vi "Construct Logging.vi"(7 "timing channel offset (-1)":i64=-1, 8 "error in":errorcluster, 10 "Logging hardware channels in":T2[](array[typedef]) {"labels settings for RT"."Label Timestamp Channel Data Reference" format="%.0x"; "labels settings for RT"."Word Initial Raw Value" format="%032.0f"; "labels settings for RT"."Label Disable/Trigger Channel Reference" format="%.0x"; "labels settings for RT"."parameter driver data"."Tx parameter refs" format="%.0x"; "labels settings for RT"."SDI" format="%02b"; "labels settings for RT"."label" format="%.0o"}, 11 "custom device ref in":T1=18446744073709551615 format="%.0x") -> (0 "error out":errorcluster, 2 "Logging Execution Unit out":refnum<class "Logging Execution Unit.lvclass">, 3 "custom device ref out":T1=18446744073709551615 format="%.0x")   [LabVIEW 2020, in "AIM ARINC 429 Engine.lvlib" / "Implementation.lvlib" / "Logging Execution Unit.lvclass"]
uses:
  Logging Execution Unit.lvclass
  Execution Unit Factory/Execution Unit Factory.lvclass
  Execution Unit/Execution Unit.lvclass
  Scripting/AIM/AIM ARINC 429 Scripting.lvlib
  C:/Users/nitest/Desktop/Git 2020/niveristand-aim-arinc429-custom-device/Source/Custom Device Support/Engine/Implementation/Execution Unit/Execution Unit.lvclass
  Shared/Label.ctl
  <vilib>/NI/NI VeriStand Encoding and Decoding/Encoding.ctl
  <vilib>/NI/NI VeriStand Encoding and Decoding/Encoding and Decoding.lvlib
  Shared/Parameter Definition.ctl
  <vilib>/NI VeriStand/Custom Device API/Custom Device Item Ref.ctl
  <vilib>/NI VeriStand/Custom Device API/Custom Device API.lvlib
  Shared/RT Parameters.ctl
  Shared/Transfer Type.ctl
  <vilib>/NI VeriStand/Custom Device API/Data Reference.ctl
  Shared/RT Label Settings.ctl
  Shared/RT Hardware Channel Settings.ctl
  Shared/Transfer Speed.ctl
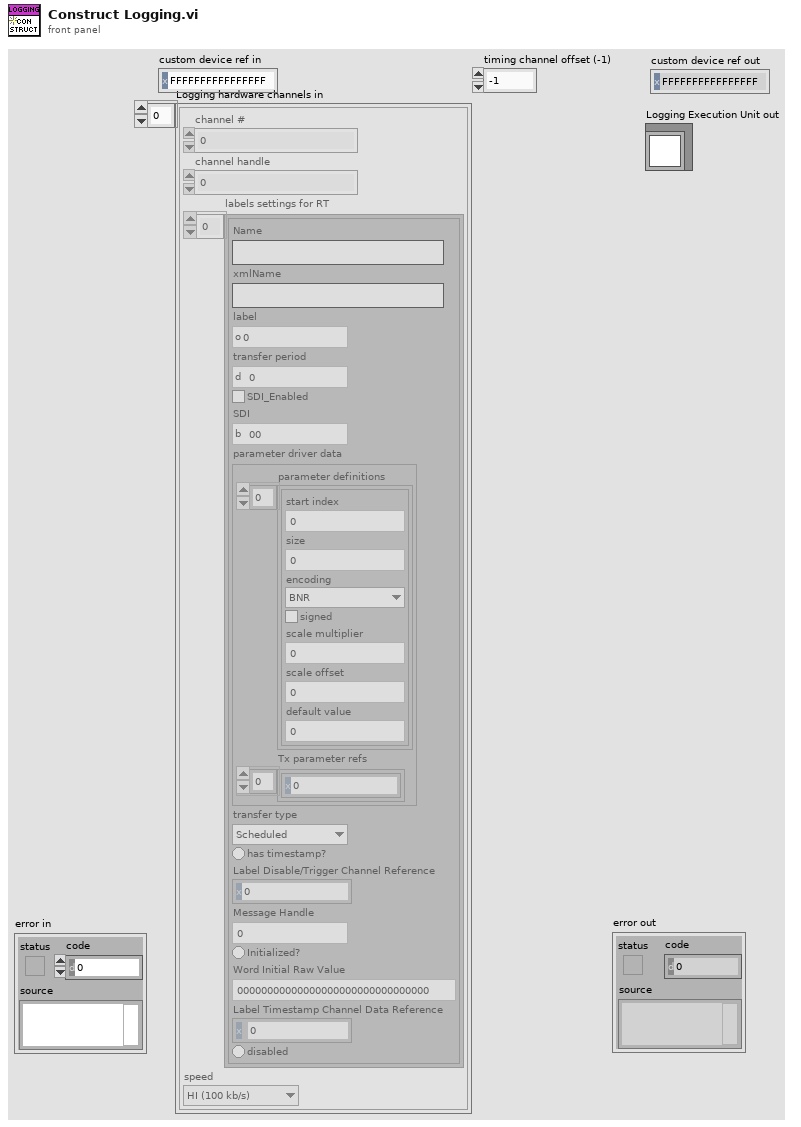
[diagram p1: front panel]
types:
  T1 = typedef "Custom Device API.lvlib/Custom Device Item Ref.ctl" = u64
  T2 = typedef "RT Hardware Channel Settings.ctl" = cluster{"channel #":u16, "channel handle":u64, "labels settings for RT":T3[], "speed":T10}
  T3 = typedef "RT Label Settings.ctl" = cluster{"Name":string, "xmlName":string, "label":T4, "transfer period":u32, "SDI_Enabled":bool, "SDI":u8, "parameter driver data":T5, "transfer type":T8, "has timestamp?":bool, "Label Disable/Trigger Channel Reference":T1, "Message Handle":u64, "Initialized?":bool, "Word Initial Raw Value":u32, "Label Timestamp Channel Data Reference":T9, "disabled":bool}
  T4 = typedef "Label.ctl" = u8
  T5 = typedef "RT Parameters.ctl" = cluster{"parameter definitions":T6[], "Tx parameter refs":T1[]}
  T6 = typedef "Parameter Definition.ctl" = cluster{"start index":i32, "size":i32, "encoding":T7, "signed":bool, "scale multiplier":dbl, "scale offset":dbl, "default value":dbl}
  T7 = typedef "Encoding and Decoding.lvlib/Encoding.ctl" = enum16{"BNR", "BCD", "Discrete"}
  T8 = typedef "Transfer Type.ctl" = enum16{"Scheduled", "Acyclic", "Block", "Strobe"}
  T9 = typedef "Custom Device API.lvlib/Data Reference.ctl" = i32
  T10 = typedef "Transfer Speed.ctl" = enum16{"LO (12.5 kb/s)", "HI (100 kb/s)"}
  T11 = typedef "Data Word Format.ctl" = string
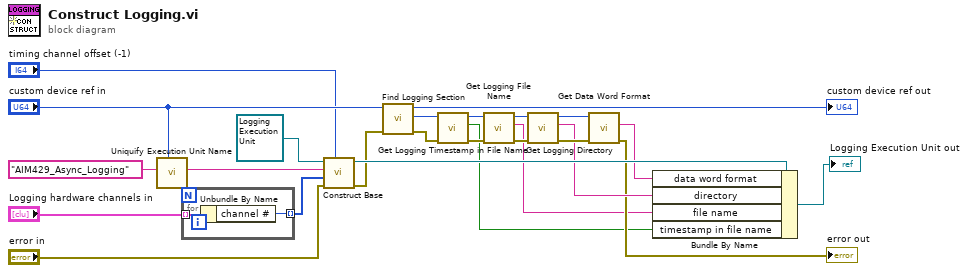
[diagram p0: block diagram]
diagram:
  n1 = call "Uniquify Execution Unit Name.vi"("custom device ref"="custom device ref in", "execution unit name"="AIM429_Async_Logging" ("identifier in")) -> ("execution unit name out"=w23:string)  [unwired: 9 in]
  n2 = for {
    tunnel: "Logging hardware channels in" -> [w27] mode=indexing
    tunnel: [w26] -> w22 mode=indexing
    n3 = Unbundle By Name(w27) -> ("channel #"=w26:u16)
  }
  n4 = call "Construct Base.vi"("timing channel offset (-1)"="timing channel offset (-1)", "error in (no error)"="error in", "channels"=w22, "identifier in"=w23, "Execution Unit in (default object)"=refnum<class "Logging Execution Unit.lvclass"> refnum ("Communication Bus Template Interfaces:Implementation.lvlib:Logging Execution Unit.lvclass")) -> ("error out"=w6:errorcluster, "Execution Unit out"=w19:refnum<class "Logging Execution Unit.lvclass">)  [unwired: 5 in]
  n5 = call "Find Logging Section.vi"("error in"=w6, "custom device ref"="custom device ref in") -> ("error out"=w5:errorcluster, "logging"=w3:T1, "custom device ref out"=→"custom device ref out":T1)  [unwired: 7 in]
  n6 = call "Get Logging Timestamp in File Name.vi"("error in"=w5, "logging ref"=w3) -> ("error out"=w18:errorcluster, "timestamp in file name"=w8:bool, "logging ref out"=w15:T1)  [unwired: 7 in]
  n7 = call "Get Logging File Name.vi"("error in"=w18, "logging ref"=w15) -> ("error out"=w17:errorcluster, "file name"=w7:string, "logging ref out"=w16:T1)  [unwired: 7 in]
  n8 = call "Get Logging Directory.vi"("error in"=w17, "logging ref"=w16) -> ("error out"=w12:errorcluster, "directory"=w11:string, "logging ref out"=w14:T1)  [unwired: 7 in]
  n9 = call "Get Data Word Format.vi"("error in"=w12, "logging ref"=w14) -> ("error out"=→"error out":errorcluster, "data word format"=w9:T11)  [unwired: 7 in, 1 out]
  n10 = Bundle By Name(cluster=w19, "data word format"=w9, "directory"=w11, "file name"=w7, "timestamp in file name"=w8) -> (→"Logging Execution Unit out":refnum<class "Logging Execution Unit.lvclass">)
